vi "ExProg_Simulate.vi"(10 "Program":T4, 11 "Simulation?":bool) -> (0 "Wanted position list":T1(array[cluster]), 1 "Used timestep (s)":sgl)   [LabVIEW 2011]
uses:
  ExperimentProgramType.ctl
  ExProgCommandType.ctl
  ExProgCommandEnumType.ctl
  Motors/MotorAxisEnum.ctl
  Motors/MotorPosType.ctl
  Typedefs/XYf.ctl
  Motors/MotorPosFlagsType.ctl
panel:
  out "loop counter":i32
  out "Instruction":i32
  in  "abort":bool
  out "FPS":dbl
  in  "Wanted Timestep (ms)":sgl=100.0
  out "Simulation Time (s)":sgl
  out "Allowed difference":T2
  # "(used for commands with string parameters)"
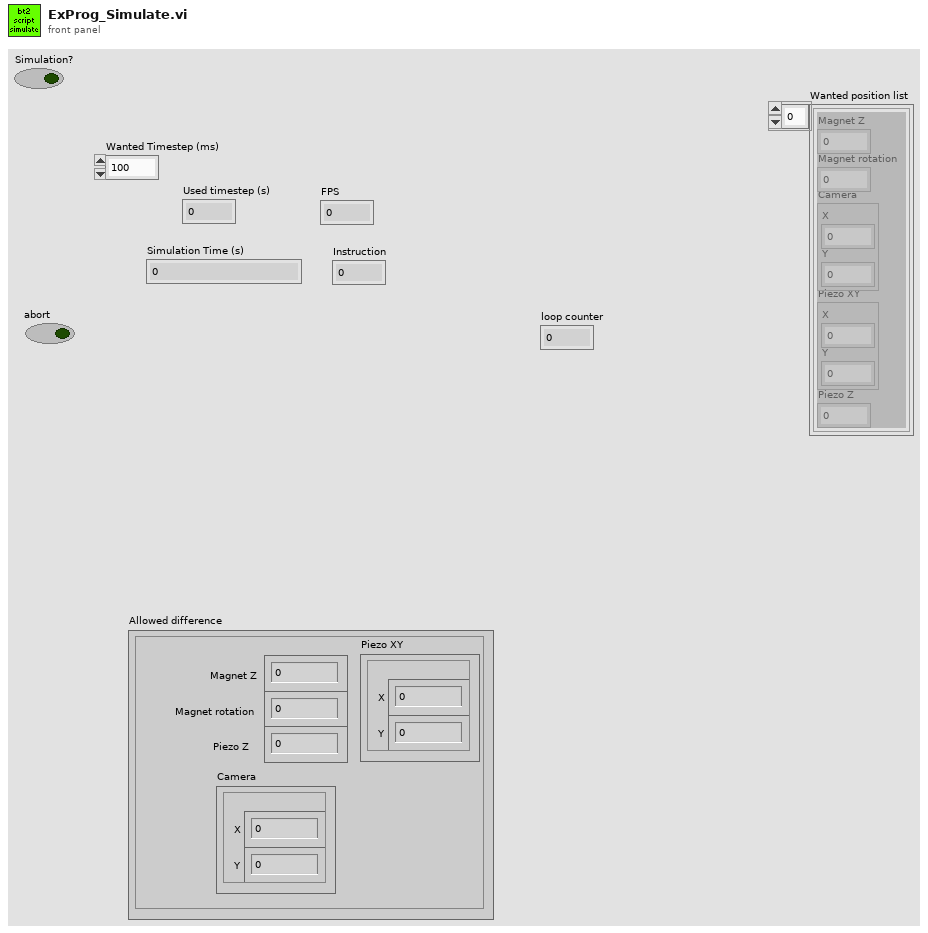
[diagram p1: front panel]
types:
  T1 = cluster{"Magnet Z":dbl, "Magnet rotation":dbl, "Camera":cluster{"X":dbl, "Y":dbl}, "Piezo XY":cluster{"X":dbl, "Y":dbl}, "Piezo Z":dbl}[]
  T2 = typedef "MotorPosType.ctl" = cluster{"Magnet Z":dbl, "Magnet rotation":dbl, "Camera":T3, "Piezo XY":T3, "Piezo Z":dbl}
  T3 = typedef "XYf.ctl" = cluster{"X":sgl, "Y":sgl}
  T4 = typedef "ExperimentProgramType.ctl" = cluster{"Commands":T5[], "Motor Axis accuracy conditions":T2, "Axis flags":T8}
  T5 = typedef "ExProgCommandType.ctl" = cluster{"cmd":T6, "axis":T7, "value/pos":dbl, "speed":dbl, "name":string}
  T6 = typedef "ExProgCommandEnumType.ctl" = enum16{"wait", "move", "acquire", "idle", "rmove", "when", "section", "stop"}
  T7 = typedef "MotorAxisEnum.ctl" = enum16{"no axis", "magrot", "magpos", "px", "py", "pz", "camx", "camy"}
  T8 = typedef "MotorPosFlagsType.ctl" = cluster{"Magnet Z":bool, "Magnet rotation":bool, "Camera":cluster{"X":bool, "Y":bool}, "Piezo XY":cluster{"X":bool, "Y":bool}, "Piezo Z":bool}
  T9 = typedef "ExProgState.ctl" = cluster{"Wanted Motorpos":T2, "Goal motorpos":T2, "Instruction":i32, "Speed":T2, "New instruction?":bool, "Instruction start time":dbl}
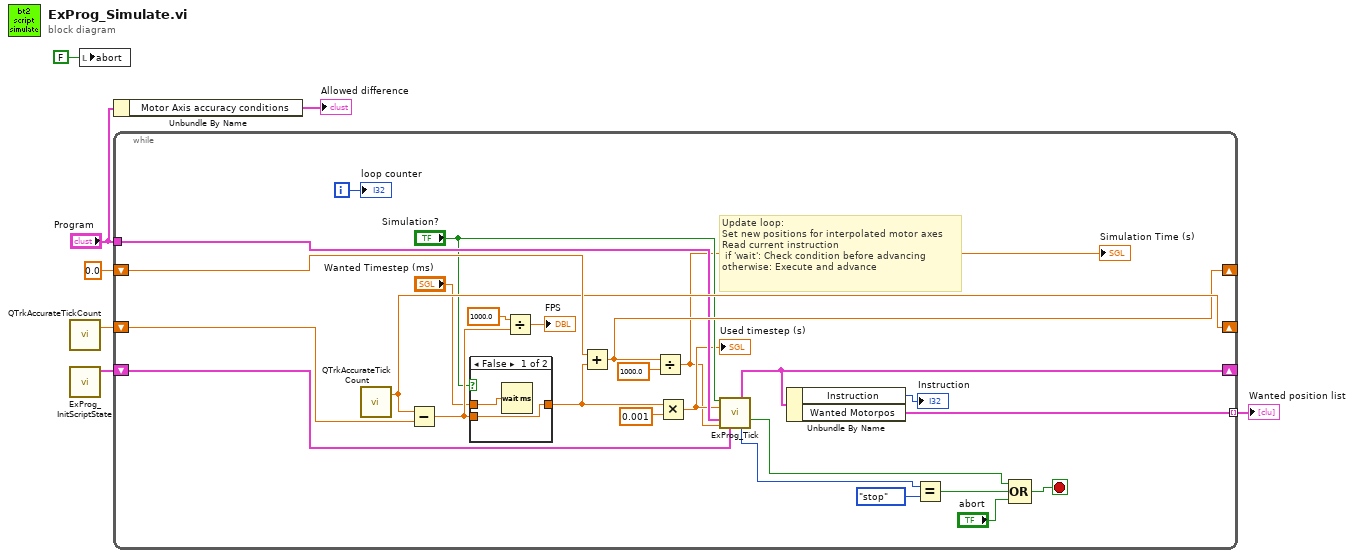
[diagram p0: block diagram]
diagram:
  n1 = call "QTrkAccurateTickCount.vi"() -> ("tick count (ms)"=w5:dbl)  [unwired: 2 in, 1 out]
  n2 = call "ExProg_InitScriptState.vi"() -> ("Script exec state out"=w1:T9)  [unwired: 11 in]
  n3 = local write "abort"(FALSE ("abort")) -> ()
  n4 = Unbundle By Name("Program") -> ("Motor Axis accuracy conditions"=→"Allowed difference":T2)
  n5 = while {
    tunnel: "Program" -> [w25]
    shift-right: [w28] -> _
    shift-left: sgl 0.0 -> [w30]
    shift-right: [w29] -> _
    shift-left: w5 -> [w33]
    tunnel: [w24] -> w4 mode=indexing
    shift-right: [w16] -> _
    shift-left: w1 -> [w17]
    i -> [w15]
    stop <- w8 stop-if-true
    # "Update loop:\nSet new positions for interpolated motor axes\nRead current instruction\n if 'wait': Check condition before advancing\notherwise: Execute and advance"
    n6 = call "QTrkAccurateTickCount.vi"() -> ("tick count (ms)"=w29:dbl)  [unwired: 2 in, 1 out]
    n7 = Subtract(x=w29, y=w33) -> (x-y=w22:dbl)
    n8 = case shown="False" "Simulation?" {
      tunnel: w22 -> [w35 _]
      tunnel: [w35 w36] -> w18
      tunnel: "Wanted Timestep (ms)" -> [w34 w36]
      frame False {
        n9 = Wait (ms)(milliseconds to wait=w34) -> ()  [unwired: 1 out]
      }
      frame True {
      }
    }
    n10 = Divide(x=1000.0, y=w22) -> (x/y=→"FPS":dbl)
    n11 = Add(x=w30, y=w18) -> (x+y=w28:dbl)
    n12 = Divide(x=w28, y=1000.0) -> (x/y=w14:dbl)
    "Simulation Time (s)" <- w14
    n13 = Multiply(x=w18, y=0.001) -> (x*y=w20:dbl)
    "Used timestep (s)" <- w20
    n14 = call "ExProg_Tick.vi"("Simulation?"="Simulation?", "Timestep (s)"=w20, "Program"=w25, "Current time (s)"=w14, "Script exec state in"=w17) -> ("Script exec state out"=w16:T9, "script ended?"=w11:bool, "Last command"=w13:T6)  [unwired: 6 in, 2 out]
    n15 = Unbundle By Name(w16) -> ("Instruction"=→"Instruction":i32, "Wanted Motorpos"=w24:T2)
    n16 = Equal?(x=w13, y=ExProgCommandEnumType."stop") -> (x = y?=w10:bool)
    n17 = Compound Arithmetic op=OR(w11, w10, "abort") -> (w8:bool)
    "loop counter" <- w15
  }
  "Wanted position list" <- w4
